vi "setUserEvent.vi"(8 "error in (no error)":errorcluster, 11 "Observer in":refnum<class "Notification.lvclass">) -> (0 "error out":errorcluster, 3 "Observer out":refnum<class "Notification.lvclass">)   [LabVIEW 2020, in "Notification.lvclass"]
uses:
  Notification.lvclass
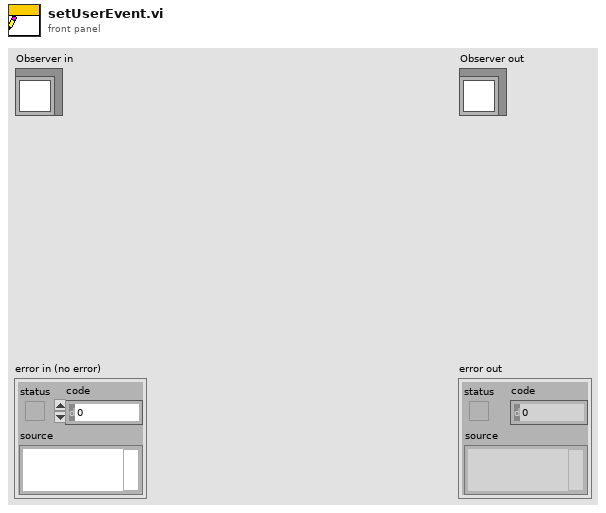
[diagram p1: front panel]
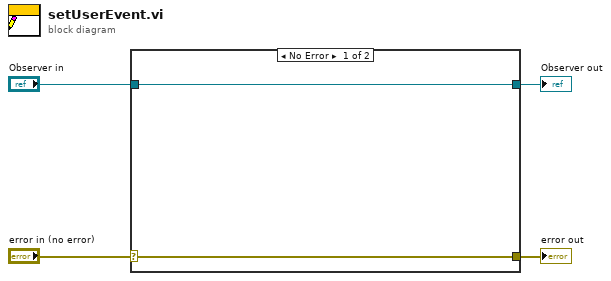
[diagram p0: block diagram]
diagram:
  n1 = case shown="No Error" "error in (no error)" {
    selector: "error in (no error)" -> [w6 w7]
    tunnel: [w6 w7] -> w3
    tunnel: [w5 w8] -> w1
    tunnel: "Observer in" -> [w5 w8]
    frame No Error {
    }
    frame Error {
    }
  }
  "error out" <- w3
  "Observer out" <- w1
